vi "Create Evaluations.vi"(8 "error in (no error)":errorcluster, 11 "IEvaluation in":refnum<class "ModeSwitch Eval.lvclass">) -> (0 "error out":errorcluster, 2 "Evaluations Out":T1[](array[typedef]) {"Low Limit" format="%#_13g"; "SI Scaling" items=["femto"=-15, "pico"=-12, "nano"=-9, "micro"=-6, "milli"=-3, "percent"=-2, ""=0, "kilo"=3, "mega"=6, "giga"=9, "tera"=12]}, 3 "IEvaluation out":refnum<class "ModeSwitch Eval.lvclass">)   [LabVIEW 2016, in "SeqAuto Evaluations.lvlib" / "ModeSwitch Eval.lvclass"]
uses:
  ModeSwitch Eval.lvclass
  C:/Sequence Automation/Plugins/SeqAuto IEvaluation.lvlibp/SeqAuto IEvaluation.lvclass
  Plugins/TestStand API Tools (TSAT).lvlibp/Evaluation Actions/Includes/Controls/TSAT Evaluation.ctl
  Plugins/TestStand API Tools (TSAT).lvlibp/Evaluation Actions/Includes/Controls/TSAT Eval SI Unit Scaling.ctl
  Plugins/TestStand API Tools (TSAT).lvlibp/Evaluation Actions/Includes/Controls/TSAT Evaluation Type.ctl
  ModeSwitch Eval.lvclass/ModeSwitch Eval.ctl
  Plugins/SeqAuto IEvaluation.lvlibp/Read Measurement Name.vi
  Plugins/TestStand API Tools (TSAT).lvlibp/Evaluation Actions/TSAT Evaluation Actions.lvlib
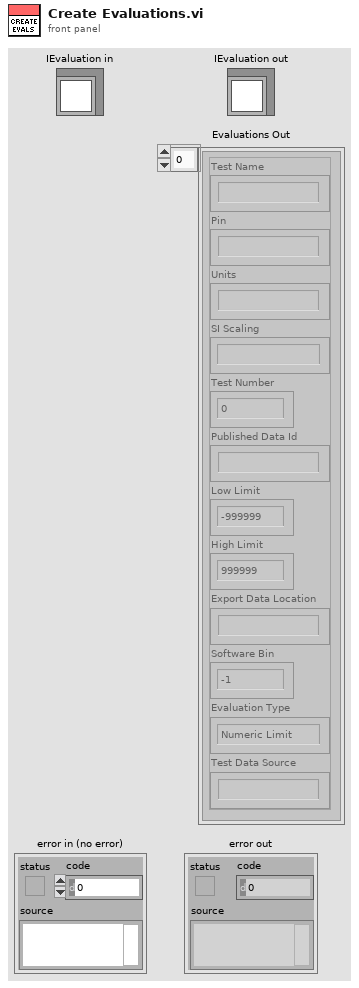
[diagram p1: front panel]
types:
  T1 = typedef "TestStand API Tools (TSAT).lvlibp/TSAT Evaluation Actions.lvlib/TSAT Evaluation.ctl" = cluster{"Test Name":string, "Pin":string, "Units":string, "SI Scaling":T2, "Test Number":i32, "Published Data Id":string, "Low Limit":dbl, "High Limit":dbl, "Export Data Location":string, "Software Bin":i64, "Evaluation Type":T3, "Test Data Source":string}
  T2 = typedef "TestStand API Tools (TSAT).lvlibp/TSAT Evaluation Actions.lvlib/TSAT Eval SI Unit Scaling.ctl" = i16
  T3 = typedef "TestStand API Tools (TSAT).lvlibp/TSAT Evaluation Actions.lvlib/TSAT Evaluation Type.ctl" = enum16{"Numeric Limit", "Pass/Fail", "None"}
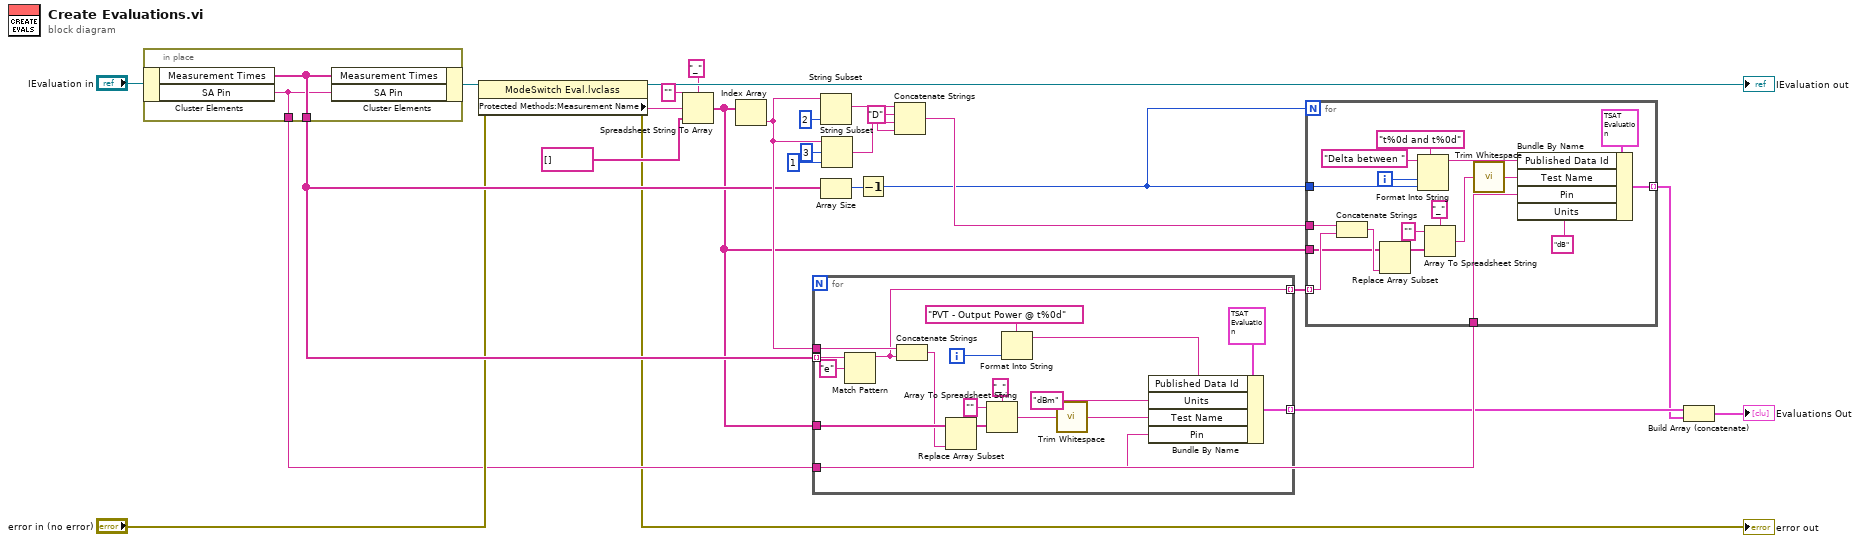
[diagram p0: block diagram]
diagram:
  w10 = "D" ("string")
  n1 = in-place {
    in-place-border: [w28] -> w15
    in-place-border: [w27] -> w5
    n2 = in-place-cluster #1("IEvaluation in") -> ("Measurement Times"=w28:string[], "SA Pin"=w27:string)
    n3 = in-place-cluster #1("Measurement Times"=w28, "SA Pin"=w27) -> (w25:refnum<class "ModeSwitch Eval.lvclass">)
  }
  n4 = property class="ModeSwitch Eval.lvclass"(reference=w25, error in="error in (no error)") -> (reference out=→"IEvaluation out":refnum<class "ModeSwitch Eval.lvclass">, error out=→"error out":errorcluster, "Protected Methods:Measurement Name"=w23:string)
  n5 = Spreadsheet String To Array(delimiter (Tab)="_", format string="", spreadsheet string=w23, array type (2D Dbl)=string[] []) -> (array=w6:string[])
  n6 = Index Array(array=w6) -> (element=w18:string)  [unwired: 1 in]
  n7 = for {
    tunnel: w15 -> [w46] mode=indexing
    tunnel: w18 -> [w44]
    tunnel: [w43] -> w13 mode=indexing
    tunnel: w6 -> [w42]
    tunnel: w5 -> [w35]
    tunnel: [w30] -> w4 mode=indexing
    i -> [w33]
    n8 = Match Pattern(string=w46, regular expression="e") -> (before substring=w43:string)  [unwired: 1 in, 3 out]
    n9 = Concatenate Strings(w44, w43) -> (w41:string)
    n10 = Replace Array Subset(array=w42, new element=w41) -> (w40:string[])  [unwired: 1 in]
    n11 = Array To Spreadsheet String(delimiter (Tab)="_", array=w40, 3:"" ("format string")) -> (spreadsheet string=w36:string)
    n12 = Format Into String(format string="PVT - Output Power @ t%0d", w33) -> (resulting string=w31:string)  [unwired: 2 in, 1 out]
    n13 = call <vilib>:"Trim Whitespace.vi"("string"=w36) -> ("trimmed string"=w29:string)  [unwired: 1 in]
    n14 = Bundle By Name(cluster=T1 {"Test Name"="", "Pin"="", "Units"="", "SI Scaling"=0, "Test Number"=0, "Published Data Id"="", "Low Limit"=-999999.0, "High Limit"=999999.0, "Export Data Location"="", "Software Bin"=-1, "Evaluation Type"=enum."Numeric Limit", "Test Data Source"=""} ("Evaluation"), "Published Data Id"=w31, "Units"="dBm", "Test Name"=w29, "Pin"=w35) -> (w30:T1)
  }
  n15 = String Subset(string=w18, length (rest)=2 ("length (rest)")) -> (substring=w12:string)  [unwired: 1 in]
  n16 = Array Size(array=w15) -> (size(s)=w14:i32)
  n17 = String Subset(string=w18, offset (0)=3, length (rest)=1 ("length (rest)")) -> (substring=w11:string)
  n18 = Decrement(x=w14) -> (x-1=w7:i32)
  n19 = Concatenate Strings(w12, w10, w11, w10) -> (w9:string)
  n20 = for {
    N: w7 -> [_]
    tunnel: w13 -> [w63] mode=indexing
    tunnel: w9 -> [w64]
    tunnel: w7 -> [w61]
    tunnel: w6 -> [w55]
    tunnel: w5 -> [w50]
    tunnel: [w48] -> w3 mode=indexing
    i -> [w62]
    n21 = Concatenate Strings(w64, w63) -> (w56:string)
    n22 = Replace Array Subset(array=w55, new element=w56) -> (w54:string[])  [unwired: 1 in]
    n23 = Format Into String(format string="t%0d and t%0d", initial string="Delta between " ("Publish ID"), w62, w61) -> (resulting string=w57:string)  [unwired: 1 in, 1 out]
    n24 = Array To Spreadsheet String(delimiter (Tab)="_", array=w54, 3:"" ("format string")) -> (spreadsheet string=w51:string)
    n25 = call <vilib>:"Trim Whitespace.vi"("string"=w51) -> ("trimmed string"=w47:string)  [unwired: 1 in]
    n26 = Bundle By Name(cluster=T1 {"Test Name"="", "Pin"="", "Units"="", "SI Scaling"=0, "Test Number"=0, "Published Data Id"="", "Low Limit"=-999999.0, "High Limit"=999999.0, "Export Data Location"="", "Software Bin"=-1, "Evaluation Type"=enum."Numeric Limit", "Test Data Source"=""} ("Evaluation"), "Published Data Id"=w57, "Test Name"=w47, "Pin"=w50, "Units"="dB") -> (w48:T1)
  }
  n27 = Build Array (concatenate)(w4, w3) -> (→"Evaluations Out":T1[])
